vi "Release UI Configuration.vi"(8 "error in (no error)":errorcluster, 11 "UIConfiguration in":refnum<class "UIConfiguration.lvclass">) -> (0 "error out":errorcluster, 3 "UIConfiguration out":refnum<class "UIConfiguration.lvclass">)   [LabVIEW 2015, in "UIConfiguration.lvclass"]
uses:
  UIConfiguration.lvclass
  UIConfiguration.lvclass/UIConfiguration.ctl
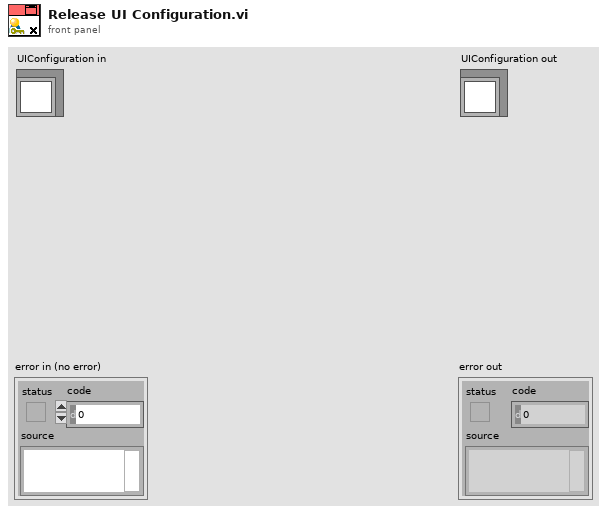
[diagram p1: front panel]
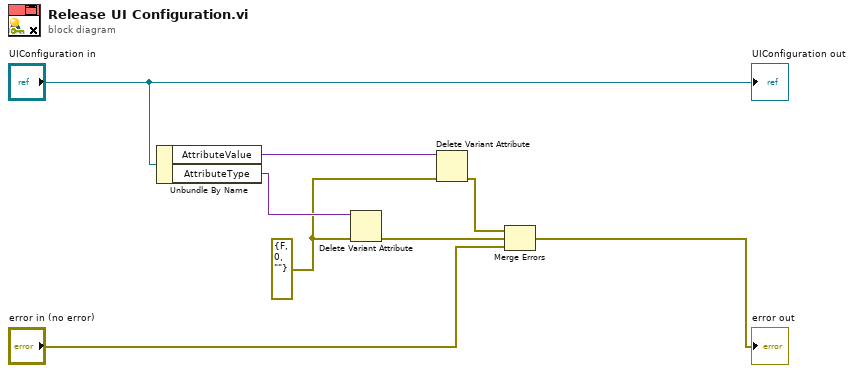
[diagram p0: block diagram]
diagram:
  w5 = errorcluster {"status"=FALSE, "code"=0, "source"=""} ("error constant")
  n1 = Unbundle By Name("UIConfiguration in") -> ("AttributeValue"=w7:variant, "AttributeType"=w6:variant)
  n2 = Delete Variant Attribute(4:w5, 7:w6) -> (0:w3:errorcluster)  [unwired: 1 in, 2 out]
  n3 = Delete Variant Attribute(4:w5, 7:w7) -> (0:w4:errorcluster)  [unwired: 1 in, 2 out]
  n4 = Merge Errors(w4, w3, "error in (no error)") -> (→"error out":errorcluster)
  "UIConfiguration out" <- "UIConfiguration in"
